vi "Program_EBN_Yann_Berton.vi"() -> ()   [LabVIEW 2020]
uses:
  Control Power/Commande.ctl
  <instrlib>/Keithley 27XX/Public/Configure/Measurement Specific/Configure Thermocouple.vi
  <instrlib>/Keithley 27XX/Public/Configure/Measurement Specific/Configure FRTD.vi
  <vilib>/Instr/_visa.llb/VISA Configure Serial Port (Instr).vi
  <instrlib>/Keithley 27XX/Keithley 27XX.lvlib
panel:
  in  "Number of samples allowed":dbl=15.0
  out "Close 50 mbar valve":bool
  out "T_ts_in_mid (wall)":dbl
  out "T_ts_in_top (wall)":dbl
  out "T_out_ts_mid (wall)":dbl
  out "T_out_ts_bot (wall)":dbl
  out "q_flux_TS (W/m²)":dbl
  out "Q_el TS (W)":dbl format="%_3g"
  out "Q_el PH (W)":dbl format="%_3g"
  in  "relative losses TS":dbl step=0.1
  in  "U Level TS":dbl step=0.1
  in  "STOP TS":bool
  out "Message 2":string
  out "Actual Voltage Level (V) TS":dbl format="%.3f"
  out "Actual Current Level (A) TS":dbl format="%.3f"
  out "status SGA":bool
  out "Power_Test section (W)":dbl format="%_3g"
  out "Warning_Temp_TS":bool
  in  "T limit_TS (C)":dbl=60.0 format="%#_13g"
  out "Temp max TS":dbl
  in  "U limit TS":dbl=8.0
  in  "I Limit TS":dbl=100.0
  out "error out 2":errorcluster caption="error out"
  in  "Power TS":bool
  out "Booléen 2":bool
  in  "relative losses PH":dbl step=0.1
  out "Counter":dbl
  out "T_PH_surf4":dbl
  out "T_PH_surf3":dbl
  out "TCHF_bot":dbl
  out "TCHF_top":dbl
  out "T3_bot":dbl
  out "T3_mid":dbl
  out "T3_top":dbl
  out "T2_top":dbl
  out "T2_mid":dbl
  out "T2_bot":dbl
  out "T1_top":dbl
  out "T1_mid":dbl
  out "T1_bot":dbl
  out "Pump cavitation":bool
  out "T_PH_surf2":dbl
  out "V_TS_corr (volts)":dbl
  out "V_PH_corr (volts)":dbl
  out "G (kg/m²s)":dbl
  out "x_out_TS":dbl
  out "x_in_TS":dbl
  out "i_in_ph":dbl
  out "i_v_TS_in":dbl
  out "i_l_TS_in":dbl
  out "T_sat(°C)":dbl
  in  "Fluid: 0 R1234ze; 1 R1233zd(E)":dbl
  out "Mass alert":bool
  in  "G minimum (kg/m²s)":dbl=20.0 format="%#_13g"
  out "Absolute pressure":dynamicdata(graph)
  out "Pressure drop":dynamicdata(graph)
  out "Temperatures":dynamicdata(graph)
  out "Temp max PH":dbl
  in  "T limit PH (C)":dbl=60.0 format="%#_13g"
  in  "STOP PH":bool
  out "Message":string
  out "Actual Voltage Level (V) PH":dbl format="%.3f"
  out "Actual Current Level (A) PH":dbl format="%.3f"
  out "Status DCS":bool
  out "Power_PRE HEATER (W)":dbl format="%_3g"
  in  "U limit PH":dbl=8.0
  in  "I Limit PH":dbl=100.0
  out "error out":errorcluster
  in  "U Level PH":dbl step=0.1
  in  "Power PH":bool
  out "Booléen":bool
  out "Warning_TEMP":bool
  in  "Porta RS232 Keithley 2701":refnum<visa-resource-name>="COM1"
  in  "Aquisition {Sample/s]":u32=1
  in  "stop":bool
  out "stop flag":bool
  out "V_TS_corr2":dbl
  out "P_reservoir (kPa)":dbl
  out "P_TS_in (kPa)":dbl
  out "P_pump_in (kPa)":dbl
  out "mass (kg/s)":dbl
  out "0-50 mbar (kPa)":dbl
  out "0-2 bar (kPa)":dbl
  out "T_ph_in (imm)":dbl
  out "T_amb":dbl
  out "T_reserv_bot":dbl
  out "T_reser_top":dbl
  out "T_TS_out_top (wall)":dbl
  out "T_TS_out (imm)":dbl
  out "T_PH_surf1":dbl
  out "T_PH_in (wall)":dbl
  out "T_TS_in (imm)":dbl
  out "T_TS_in_bot (wall)":dbl
  out "T_pump_in":dbl
  in  "File":path=path "C:/test.lvm" caption="Filename"
  in  "Save":bool caption="Enable"
  out "0-5 bar (kPa)":dbl
  out "Tcj ch201":dbl
  # "SAVING DATA"
  # "SGA Power supply: TEST SECTION POWER"
  # "DCS Power supply: PRE-HEATER POWER"
  # "Pre-heater temperatures"
  # "Test section temperatures"
  # "85 mm mm"
  # "40 mm"
  # "62.5 mm mm"
  # "665 mm"
  # "1347 mm mm"
  # "115 mm mm"
  # "809 mm"
  # "1585 mm mm"
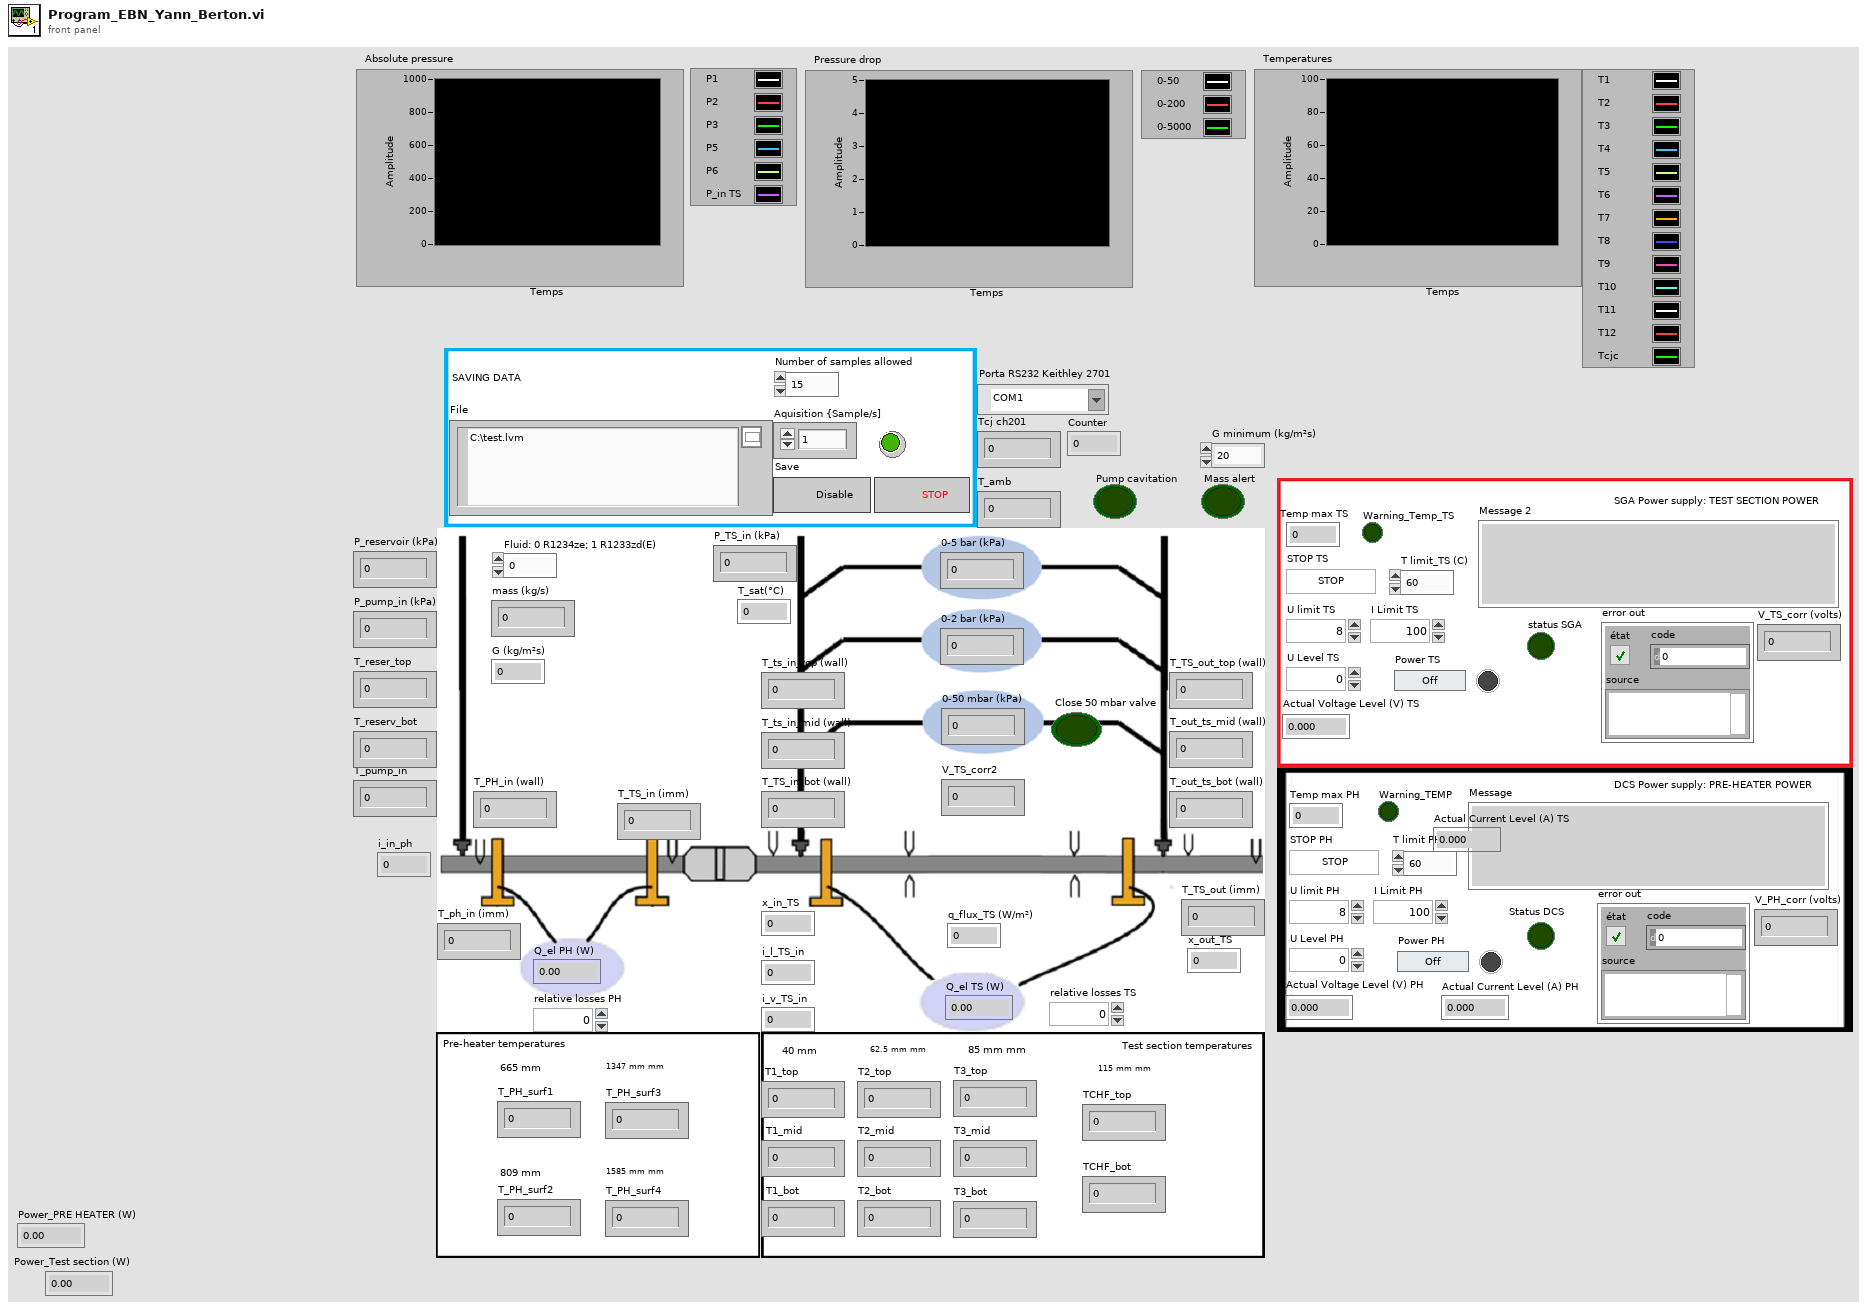
[diagram p1: front panel]
types:
  T1 = typedef "Commande.ctl" = enum16{"Power ON/OFF", "WaitForEvent", "Limit U&I", "Send ui", "Send U", "Meas", "Stop", "Init"}
  T2 = cluster{"Baud Rate (9600)":u32, "Flow Control (1: XON/XOFF)":u16, "Termination Char (0:CR)":u16}
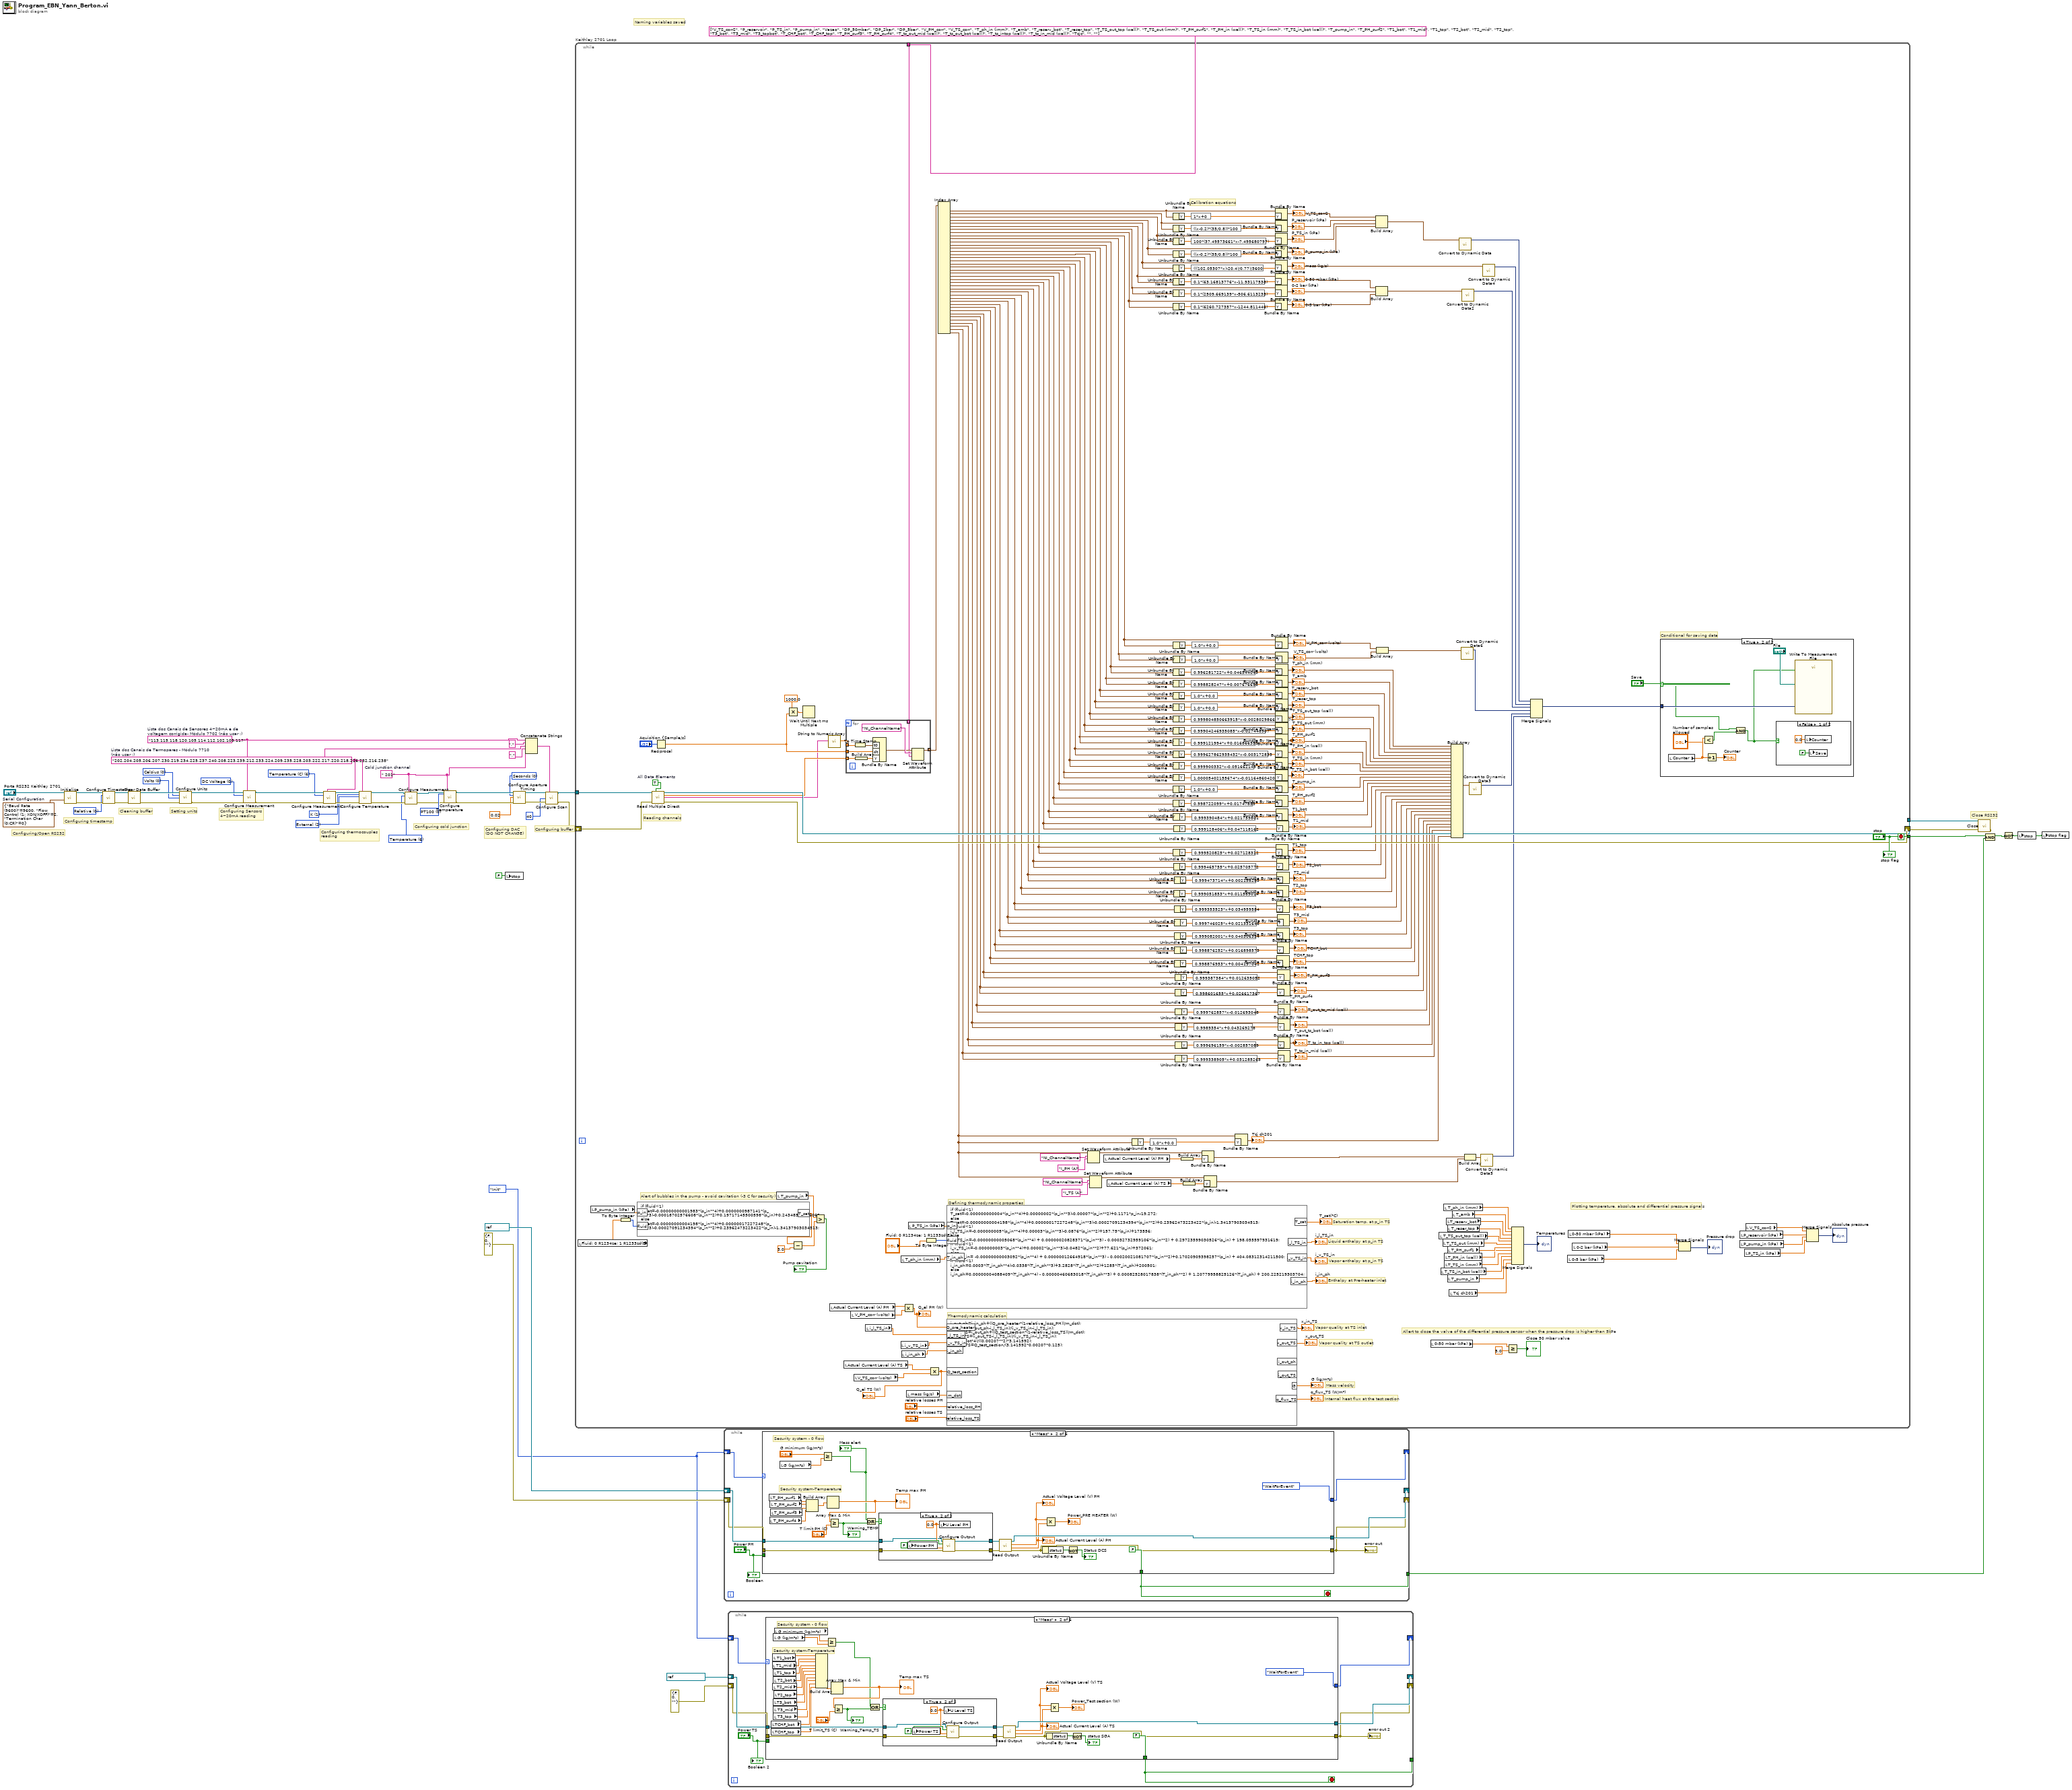
[diagram p0: block diagram]
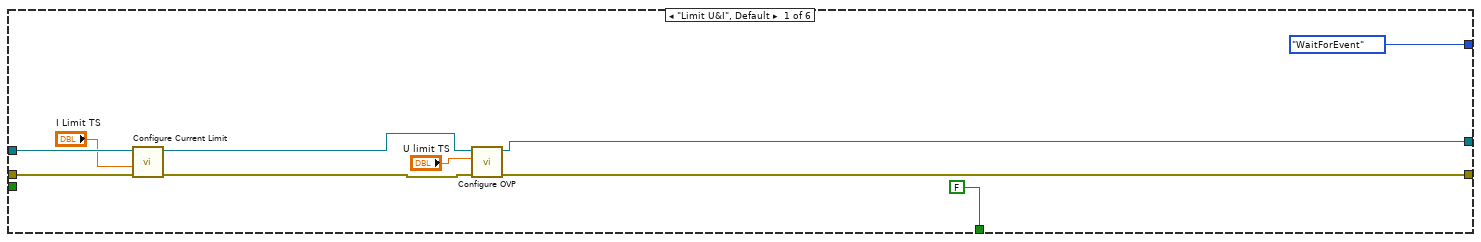
[diagram p2: hidden frame]
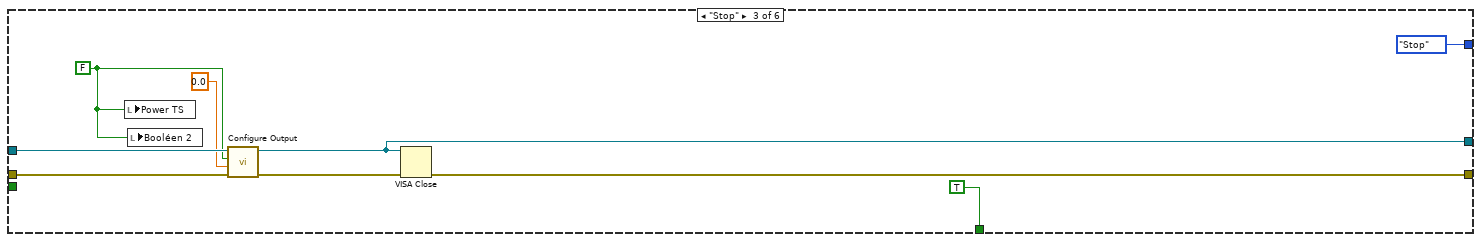
[diagram p4: hidden frame]
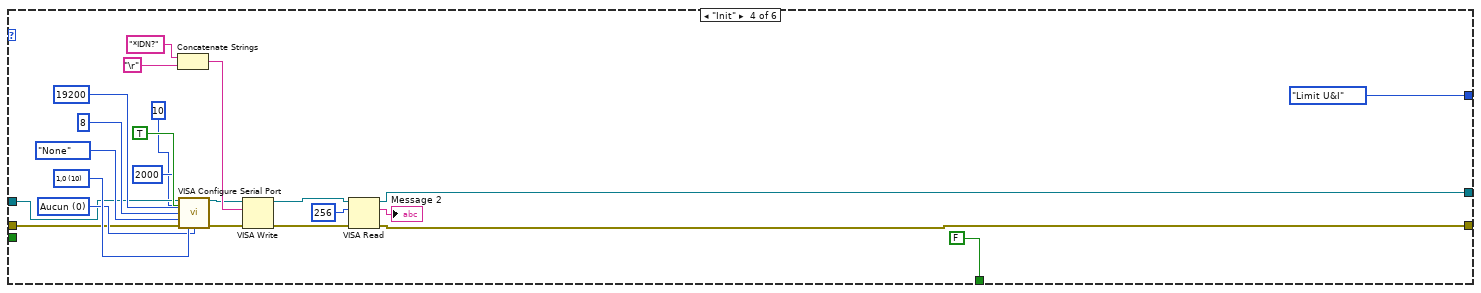
[diagram p5: hidden frame]
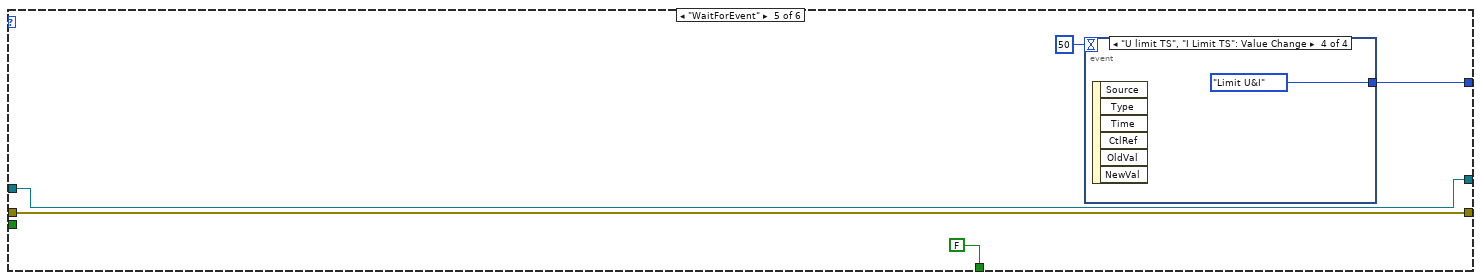
[diagram p6: hidden frame]
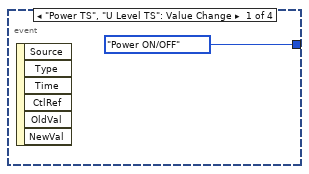
[diagram p7: hidden frame]
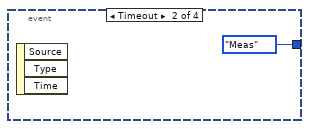
[diagram p8: hidden frame]
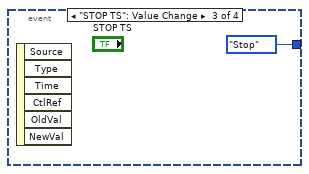
[diagram p9: hidden frame]
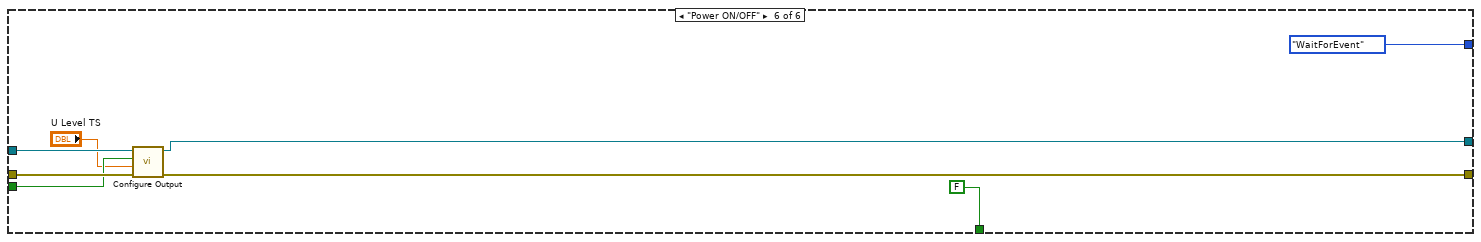
[diagram p10: hidden frame]
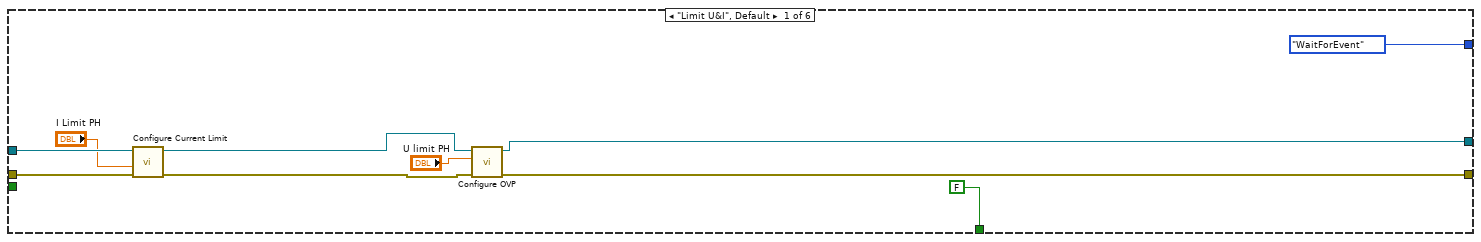
[diagram p11: hidden frame]
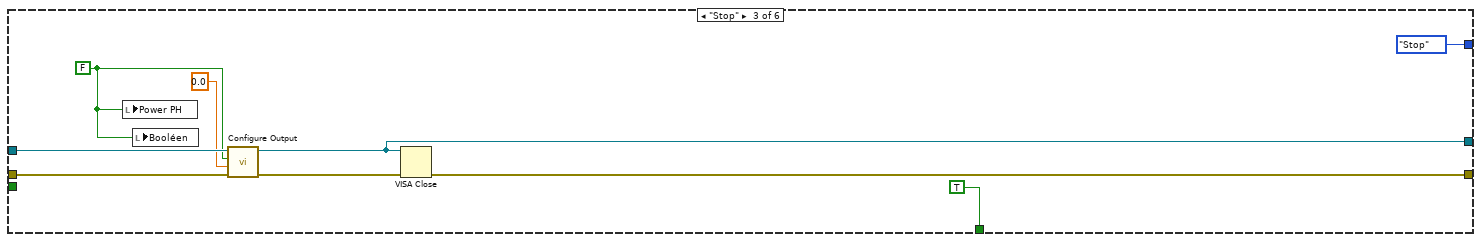
[diagram p13: hidden frame]
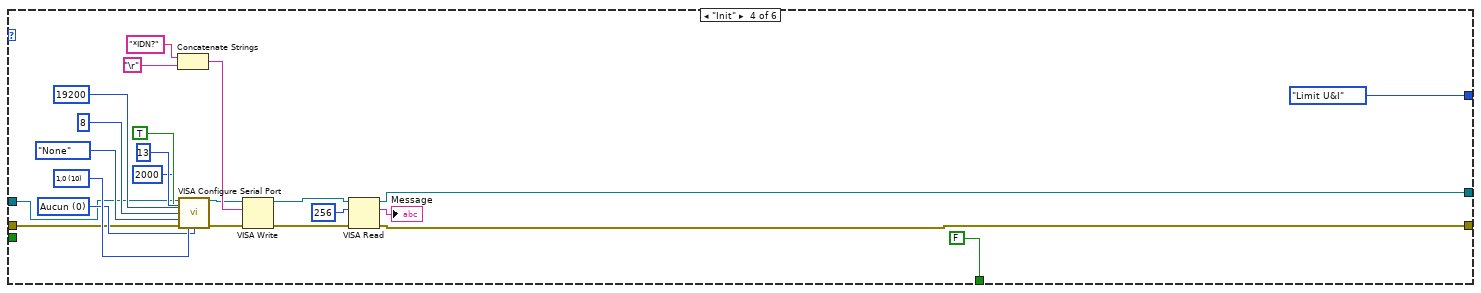
[diagram p14: hidden frame]
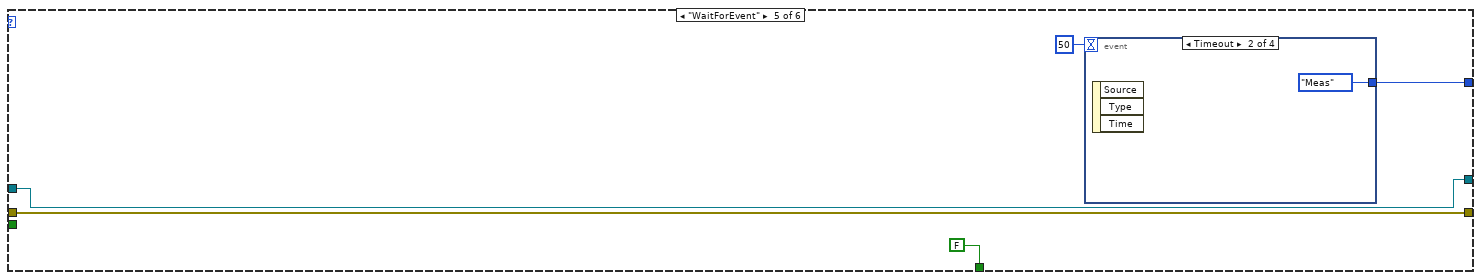
[diagram p15: hidden frame]
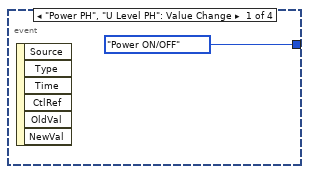
[diagram p16: hidden frame]
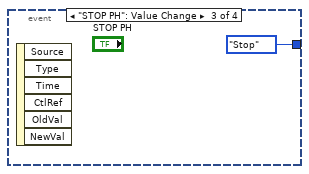
[diagram p17: hidden frame]
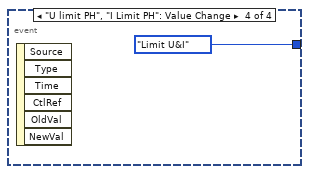
[diagram p18: hidden frame]
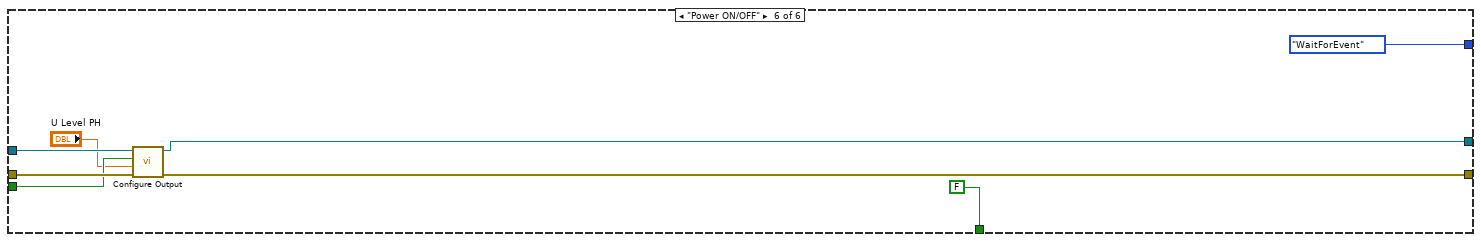
[diagram p19: hidden frame]
diagram:
  w3 = Commande."Init"
  w23 = u16 0 items=["PT100", "D100", "F100", "PT3916", "PT385", "USER"] ("FRTD Type (0: PT100)")
  w26 = u16 6 items=["DC Voltage", "AC Voltage", "DC Current", "AC Current", "Resistance", "Four-Wire Resistance", "Temperature", "Frequency", "Period", "Continuity"] ("Function (0: DC Voltage)")
  w24 = " 201"  # Cold junction channel
  w32 = "202,204,205,206,207,230,219,234,225,237,240,208,223,239,212,233,224,209,235,228,203,222,217,220,218,226,232,216,238"  # Lista dos Canais de Termopares - Módulo 7710 (não usar :)
  w40 = "113,115,118,120,105,114,112,102,109,117"  # Lista dos Canais de Sensores 4~20mA e de voltagem corrigida- Módulo 7702 (não usar :)
  w19 = u16 0 items=["Seconds", "Power Line Cycles"] ("Timing Units (0: Seconds)")
  w29 = u16 2 items=["Simulated", "Internal", "External"] ("Reference Junction Type (0: Simulated)")
  w30 = u16 1 items=["J", "K", "T", "E", "R", "S", "B", "N"] ("Thermocouple Type (1: K)")
  w41 = u16 0 items=["Volts", "dB"] ("DC Voltage (0: V)")
  w42 = u16 0 items=["Celsius", "Fahrenheit", "Kelvin"] ("Temperature (0: Celsius)")
  w34 = u16 6 items=["DC Voltage", "AC Voltage", "DC Current", "AC Current", "Resistance", "Four-Wire Resistance", "Temperature (C)", "Frequency", "Period", "Continuity"] ("Function (0: DC Voltage)")
  w37 = u16 0 items=["DC Voltage", "AC Voltage", "DC Current", "AC Current", "Resistance", "Four-Wire Resistance", "Temperature (C)", "Frequency", "Period", "Continuity"] ("Function (0: DC Voltage)")
  w50 = T2 {"Baud Rate (9600)"=9600, "Flow Control (1: XON/XOFF)"=2, "Termination Char (0:CR)"=0}  # Serial Configuration
  w47 = u16 0 items=["Relative", "Real Time Clock"] ("Timestamp Type (0: Relative)")
  # "Configuring cold junction"
  # "Naming variables saved"
  # "Close RS232"
  # "Configuring buffer"
  # "Configuring DAC \n(DO NOT CHANGE)"
  # "Configuring thermocouples\nreading"
  # "Configuring Sensors \n4~20mA reading"
  # "Setting units"
  # "Cleaning buffer"
  # "Configuring timestamp"
  # "Configuring/Open RS232"
  n1 = call <instrlib>:"Initialize.vi"("VISA resource name"="Porta RS232 Keithley 2701", "Serial Configuration"=w50) -> ("VISA resource name out"=w49:refnum<visa-resource-name>, "error out"=w48:errorcluster)  [unwired: 12 in]
  n2 = call <instrlib>:"Configure Timestamp.vi"("VISA resource name"=w49, "Timestamp Type (0: Relative)"=w47, "error in (no error)"=w48) -> ("VISA resource name out"=w46:refnum<visa-resource-name>, "error out"=w45:errorcluster)  [unwired: 11 in]
  n3 = call <instrlib>:"Clear Data Buffer.vi"("VISA resource name"=w46, "error in (no error)"=w45) -> ("VISA resource name out"=w44:refnum<visa-resource-name>, "error out"=w43:errorcluster)  [unwired: 12 in]
  n4 = call <instrlib>:"Configure Units.vi"("VISA resource name"=w44, "Temperature (0: Celsius)"=w42, "DC Voltage (0: V)"=w41, "error in (no error)"=w43) -> ("VISA resource name out"=w38:refnum<visa-resource-name>, "error out"=w39:errorcluster)  [unwired: 10 in]
  n5 = call <instrlib>:"Configure Measurement.vi"("VISA resource name"=w38, "Scan List (Empty)"=w40, "Function (0: DC Voltage)"=w37, "error in (no error)"=w39) -> ("VISA resource name out"=w36:refnum<visa-resource-name>, "error out"=w35:errorcluster)  [unwired: 10 in]
  n6 = call <instrlib>:"Configure Measurement.vi"("VISA resource name"=w36, "Scan List (Empty)"=w32, "Function (0: DC Voltage)"=w34, "error in (no error)"=w35) -> ("VISA resource name out"=w33:refnum<visa-resource-name>, "error out"=w31:errorcluster)  [unwired: 10 in]
  n7 = call-poly <instrlib>:"Configure Temperature.vi"("VISA resource name"=w33, "Thermocouple Type (1: K)"=w30, "Reference Junction Type (0: Simulated)"=w29, "error in (no error)"=w31, "Scan List (Empty)"=w32) -> ("VISA resource name out"=w28:refnum<visa-resource-name>, "error out"=w27:errorcluster)  [unwired: 13 in]
  n8 = call <instrlib>:"Configure Measurement.vi"("VISA resource name"=w28, "Scan List (Empty)"=w24, "Function (0: DC Voltage)"=w26, "error in (no error)"=w27) -> ("VISA resource name out"=w25:refnum<visa-resource-name>, "error out"=w22:errorcluster)  [unwired: 10 in]
  n9 = call-poly <instrlib>:"Configure Temperature.vi"("VISA resource name"=w25, "FRTD Type (0: PT100)"=w23, "error in (no error)"=w22, "Scan List (Empty)"=w24) -> ("VISA resource name out"=w21:refnum<visa-resource-name>, "error out"=w20:errorcluster)  [unwired: 14 in]
  n10 = local write "stop"(FALSE ("stop")) -> ()
  n11 = call <instrlib>:"Configure Aperture Timing.vi"("VISA resource name"=w21, "Timing Units (0: Seconds)"=w19, "Timing Value (0.020)"=0.02, "error in (no error)"=w20) -> ("VISA resource name out"=w16:refnum<visa-resource-name>, "error out"=w15:errorcluster)  [unwired: 10 in]
  n12 = Concatenate Strings(w40, "," ("string"), w32, "," ("string"), w24) -> (w17:string)
  n13 = call <instrlib>:"Configure Scan.vi"("VISA resource name"=w16, "Channel List (101:110)"=w17, "Sample Count (100)"=40 ("Sample Count (10)"), "error in (no error)"=w15) -> ("VISA resource name out"=w13:refnum<visa-resource-name>, "error out"=w14:errorcluster)  [unwired: 10 in]
  n14 = while "Keithley 2701 Loop" {
    tunnel: w13 -> [w257]
    tunnel: [w254] -> w11
    shift-right: [w255] -> w10
    shift-left: w14 -> [w256]
    tunnel: string[] ["V_TS_corr2", "P_reservoir", "P_TS_in", "P_pump_in", "Vazao", "DP_50mbar", "DP_2bar", "DP_5bar", "V_PH_corr", "V_TS_corr", "T_ph_in (imm)", "T_amb", "T_reserv_bot", "T_reser_top", "T_TS_out_top (wall)", "T_TS_out (imm)", "T_PH_surf1", "T_PH_in (wall)", "T_TS_in (imm)", "T_TS_in_bot (wall)", "T_pump_in", "T_PH_surf2", "T1_bot", "T1_mid", "T1_top", "T2_bot", "T2_mid", "T2_top", "T3_bot", "T3_mid", "T3_topbot", "T_CHF_bot", "T_CHF_top", "T_PH_surf3", "T_PH_surf4", "T_ts_out_mid (wall)", "T_ts_out_bot (wall)", "T_ts_intop (wall)", "T_ts_in_mid (wall)", "Tcjc", "", ""] -> [w308]
    tunnel: ["stop"] -> w7
    stop <- "stop" stop-if-true
    w250 = TRUE  # All Data Elements
    # "Allert to close the valve of the differential pressure sensor when the pressure drop is higher than 5kPa"
    # "Internal heat flux at the test section"
    # "Alert of bubbles in the pump - avoid cavitation (-3 C for security)"
    # "Mass velocity"
    # "Vapor quality at TS outlet"
    # "Vapor quality at TS inlet"
    # "Thermodynamic calculation"
    # "Enthalpy at Pre-heater inlet"
    # "Vapor enthalpy at p_in TS"
    # "Liquid enthalpy at p_in TS"
    # "Saturation temp. at p_in TS"
    # "Defining thermodynamic properties"
    # "Plotting temperature, absolute and differential pressure signals"
    # "Conditional for saving data"
    # "Calibration equations"
    # "Reading channels"
    n15 = local read "Fluid: 0 R1234ze; 1 R1233zd(E)"() -> (w166:dbl)
    n16 = local read "P_pump_in (kPa)"() -> (w172:dbl)
    n17 = To Byte Integer(number=w166) -> (8bit integer=w165:i8)
    n18 = formula code="if (fluid<1)\nT_sat=-0.00000000001983*(p_in**4)+0.0000000987141*(p_in**3)-0.00018702576608*(p_in**2)+0.19717145500598*(p_in)+0.24348535016065;\nelse\nT_sat=-0.00000000004198*(p_in**4)+0.00000017227248*(p_in**3)-0.00027091234394*(p_in**2)+0.23962473223422*(p_in)-1.34137903034513;"("p_in"=w172, "fluid"=w165) -> ("T_sat"=w168:dbl)
    n19 = call <instrlib>:"Read Multiple Direct.vi"("VISA resource name"=w257, "All Data Elements (False)"=w250, "error in (no error)"=w256) -> ("VISA resource name out"=w254:refnum<visa-resource-name>, "Measurement Data"=w253:dbl[], "Time Stamp"=w252:string[], "error out"=w255:errorcluster)  [unwired: 7 in, 2 out]
    n20 = Reciprocal(x="Aquisition {Sample/s]") -> (1/x=w309:dbl)
    n21 = local read "T_pump_in"() -> (w171:dbl)
    n22 = Multiply(x=1000.0 ("y"), y=w309) -> (x*y=w310:dbl)
    n23 = Subtract(x=w168, y=3.0) -> (x-y=w167:dbl)
    n24 = Wait Until Next ms Multiple(millisecond multiple=w310) -> ()  [unwired: 1 out]
    n25 = Greater?(x=w171, y=w167) -> (0:→"Pump cavitation":bool)
    n26 = call <instrlib>:"String to Numeric Array.vi"("String Array"=w252) -> ("Numeric Array"=w251:dbl[])  [unwired: 10 in]
    n27 = local read "Actual Current Level (A) PH"() -> (w89:dbl)
    n28 = local read "Actual Current Level (A) TS"() -> (w85:dbl)
    n29 = for {
      tunnel: w251 -> [w331] mode=indexing
      tunnel: w253 -> [w329] mode=indexing
      tunnel: w309 -> [w327]
      tunnel: w308 -> [w324] mode=indexing
      tunnel: [w323] -> w307 mode=indexing
      n30 = To Time Stamp(1:w331) -> (0:w330:timestamp)
      n31 = Build Array(w329) -> (w328:dbl[])
      n32 = Bundle By Name("t0"=w330, "dt"=w327, "Y"=w328) -> (w325:waveform(dbl))  [unwired: 1 in]
      n33 = Set Waveform Attribute(5:w324, 6:"NI_ChannelName" ("name"), 7:w325) -> (3:w323:waveform(dbl))  [unwired: 1 in, 2 out]
    }
    n34 = local read "V_PH_corr (volts)"() -> (w88:dbl)
    n35 = local read "V_TS_corr (volts)"() -> (w86:dbl)
    n36 = local read "i_l_TS_in"() -> (w58:dbl)
    n37 = local read "i_v_TS_in"() -> (w57:dbl)
    n38 = local read "T_ph_in (imm)"() -> (w212:dbl)
    n39 = local read "i_in_ph"() -> (w56:dbl)
    n40 = Multiply(x=w89, y=w88) -> (x*y=w87:dbl)
    "Q_el PH (W)" <- w87
    n41 = local read "mass (kg/s)"() -> (w164:dbl)
    n42 = local read "P_TS_in (kPa)"() -> (w214:dbl)
    n43 = To Byte Integer(number="Fluid: 0 R1234ze; 1 R1233zd(E)") -> (8bit integer=w205:i8)
    n44 = Multiply(x=w85, y=w86) -> (x*y=w83:dbl)
    "Q_el TS (W)" <- w83
    n45 = Index Array(array=w307) -> (element #1=w200:waveform(dbl), element #2=w199:waveform(dbl), element #3=w198:waveform(dbl), element #4=w197:waveform(dbl), element #5=w196:waveform(dbl), element #6=w195:waveform(dbl), element #7=w61:waveform(dbl), element #8=w194:waveform(dbl), element #9=w186:waveform(dbl), element #10=w183:waveform(dbl), element #11=w262:waveform(dbl), element #12=w263:waveform(dbl), element #13=w264:waveform(dbl), element #14=w265:waveform(dbl), element #15=w266:waveform(dbl), element #16=w267:waveform(dbl), element #17=w268:waveform(dbl), element #18=w269:waveform(dbl), element #19=w270:waveform(dbl), element #20=w271:waveform(dbl), element #21=w272:waveform(dbl), element #22=w173:waveform(dbl), element #23=w161:waveform(dbl), element #24=w156:waveform(dbl), element #25=w155:waveform(dbl), element #26=w148:waveform(dbl), element #27=w147:waveform(dbl), element #28=w146:waveform(dbl), element #29=w139:waveform(dbl), element #30=w138:waveform(dbl), element #31=w137:waveform(dbl), element #32=w132:waveform(dbl), element #33=w131:waveform(dbl), element #34=w94:waveform(dbl), element #35=w93:waveform(dbl), element #36=w77:waveform(dbl), element #37=w76:waveform(dbl), element #38=w71:waveform(dbl), element #39=w67:waveform(dbl), element #40=w59:waveform(dbl))  [unwired: 40 in]
    n46 = formula code="if (fluid<1)\nT_sat=-0.000000000004*(p_in**4)+0.00000002*(p_in**3)-0.00007*(p_in**2)+0.1171*p_in-19.272;\nelse\nT_sat=-0.00000000004198*(p_in**4)+0.00000017227248*(p_in**3)-0.00027091234394*(p_in**2)+0.23962473223422*(p_in)-1.34137903034513;\nif (fluid<1)\ni_l_TS_in=-0.000000005*(p_in**4)+0.00003*(p_in**3)-0.0876*(p_in**2)+157.75*(p_in)+173556;\nelse\ni_l_TS_in=-0.00000000005068*(p_in**4) + 0.00000020828371*(p_in**3) - 0.00032732959106*(p_in**2) + 0.29723599030526*(p_in) + 198.055597931619;\nif (fluid<1)\ni_v_TS_in=-0.000000003*(p_in**4)+0.00002*(p_in**3)-0.0482*(p_in**2)+77.621*(p_in)+372061;\nelse \ni_v_TS_in= -0.00000000003092*(p_in**4) + 0.00000012664918*(p_in**3) - 0.00020021081707*(p_in**2)+0.17020909398257*(p_in) + 404.08312314211500;\nif (fluid<1)\ni_in_ph=0.0003*(T_in_ph**4)-0.0338*(T_in_ph**3)+3.2828*(T_in_ph**2)+1285*(T_in_ph)+200501;\nelse\ni_in_ph=0.00000004088409*(T_in_ph**4) - 0.00000460683018*(T_in_ph**3) + 0.00082528017838*(T_in_ph**2) + 1.20779958825126*(T_in_ph) + 200.225219303704;"("p_in"=w214, "fluid"=w205, "T_in_ph"=w212) -> ("T_sat"=→"T_sat(°C)":dbl, "i_l_TS_in"=→"i_l_TS_in":dbl, "i_v_TS_in"=→"i_v_TS_in":dbl, "i_in_ph"=→"i_in_ph":dbl)
    n47 = formula code="i_out_ph=i_in_ph+((Q_pre_heater*(1-relative_loss_PH))/m_dot);\nx_in_TS=(i_out_ph-i_l_TS_in)/(i_v_TS_in-i_l_TS_in);\ni_out_TS=i_out_ph+((Q_test_section*(1-relative_loss_TS))/m_dot);\nx_out_TS=(i_out_TS-i_l_TS_in)/(i_v_TS_in-i_l_TS_in);\nG=(m_dot*4)/((0.00207**2)*3.141592);\nq_flux_TS=Q_test_section/(3.141592*0.00207*0.125);"("i_l_TS_in"=w58, "i_v_TS_in"=w57, "i_in_ph"=w56, "Q_pre_heater"=w87, "Q_test_section"=w83, "m_dot"=w164, "relative_loss_PH"="relative losses PH", "relative_loss_TS"="relative losses TS") -> ("x_in_TS"=→"x_in_TS":dbl, "x_out_TS"=→"x_out_TS":dbl, "G"=→"G (kg/m²s)":dbl, "q_flux_TS"=→"q_flux_TS (W/m²)":dbl)  [unwired: 2 out]
    n48 = Set Waveform Attribute(5:"I_PH (A)" ("name"), 6:"NI_ChannelName" ("name"), 7:w59) -> (3:w247:waveform(dbl))  [unwired: 1 in, 2 out]
    n49 = Set Waveform Attribute(5:"I_TS (A)" ("name"), 6:"NI_ChannelName" ("name"), 7:w59) -> (3:w102:waveform(dbl))  [unwired: 1 in, 2 out]
    n50 = local read "Actual Current Level (A) PH"() -> (w177:dbl)
    n51 = local read "Actual Current Level (A) TS"() -> (w104:dbl)
    n52 = Unbundle By Name(w59) -> ("Y"=w261:dbl[])
    n53 = expression code="1.0*x+0.0"(w261) -> (w232:dbl[])
    n54 = Unbundle By Name(w200) -> ("Y"=w305:dbl[])
    n55 = Unbundle By Name(w199) -> ("Y"=w302:dbl[])
    n56 = Unbundle By Name(w198) -> ("Y"=w304:dbl[])
    n57 = Unbundle By Name(w197) -> ("Y"=w297:dbl[])
    n58 = Unbundle By Name(w196) -> ("Y"=w301:dbl[])
    n59 = Unbundle By Name(w195) -> ("Y"=w298:dbl[])
    n60 = Unbundle By Name(w61) -> ("Y"=w295:dbl[])
    n61 = Unbundle By Name(w194) -> ("Y"=w274:dbl[])
    n62 = Unbundle By Name(w262) -> ("Y"=w293:dbl[])
    n63 = Unbundle By Name(w263) -> ("Y"=w291:dbl[])
    n64 = Unbundle By Name(w264) -> ("Y"=w292:dbl[])
    n65 = Unbundle By Name(w265) -> ("Y"=w287:dbl[])
    n66 = Unbundle By Name(w266) -> ("Y"=w288:dbl[])
    n67 = Unbundle By Name(w267) -> ("Y"=w290:dbl[])
    n68 = Unbundle By Name(w268) -> ("Y"=w289:dbl[])
    n69 = Unbundle By Name(w269) -> ("Y"=w283:dbl[])
    n70 = Unbundle By Name(w270) -> ("Y"=w286:dbl[])
    n71 = Unbundle By Name(w271) -> ("Y"=w285:dbl[])
    n72 = Unbundle By Name(w272) -> ("Y"=w284:dbl[])
    n73 = Unbundle By Name(w173) -> ("Y"=w175:dbl[])
    n74 = Unbundle By Name(w186) -> ("Y"=w188:dbl[])
    n75 = Unbundle By Name(w183) -> ("Y"=w184:dbl[])
    n76 = Unbundle By Name(w161) -> ("Y"=w162:dbl[])
    n77 = Unbundle By Name(w155) -> ("Y"=w157:dbl[])
    n78 = Unbundle By Name(w156) -> ("Y"=w160:dbl[])
    n79 = Unbundle By Name(w148) -> ("Y"=w154:dbl[])
    n80 = Unbundle By Name(w146) -> ("Y"=w150:dbl[])
    n81 = Unbundle By Name(w147) -> ("Y"=w152:dbl[])
    n82 = Unbundle By Name(w139) -> ("Y"=w140:dbl[])
    n83 = Unbundle By Name(w137) -> ("Y"=w144:dbl[])
    n84 = Unbundle By Name(w131) -> ("Y"=w134:dbl[])
    n85 = Unbundle By Name(w138) -> ("Y"=w142:dbl[])
    n86 = Unbundle By Name(w132) -> ("Y"=w136:dbl[])
    n87 = Unbundle By Name(w94) -> ("Y"=w98:dbl[])
    n88 = Unbundle By Name(w93) -> ("Y"=w96:dbl[])
    n89 = Unbundle By Name(w77) -> ("Y"=w78:dbl[])
    n90 = Unbundle By Name(w76) -> ("Y"=w80:dbl[])
    n91 = Unbundle By Name(w71) -> ("Y"=w73:dbl[])
    n92 = Unbundle By Name(w67) -> ("Y"=w68:dbl[])
    n93 = Build Array(w177) -> (w246:dbl[])
    n94 = Build Array(w104) -> (w103:dbl[])
    n95 = expression code="1*x+0"(w305) -> (w306:dbl[])
    n96 = expression code="((x-0.2)*(35/0.8))*100"(w302) -> (w303:dbl[])
    n97 = expression code="100*(37.49573661*x-7.495680797)"(w304) -> (w260:dbl[])
    n98 = expression code="((x-0.2)*(35/0.8))*100"(w297) -> (w296:dbl[])
    n99 = expression code="(((102.05307*x)-20.4)/0.77)/3600"(w301) -> (w300:dbl[])
    n100 = expression code="0.1*(63.16813776*x-11.93117538)"(w298) -> (w299:dbl[])
    n101 = expression code="0.1*(2509.669139*x-506.6113235)"(w295) -> (w294:dbl[])
    n102 = expression code="0.1*(6260.727357*x-1244.811446)"(w274) -> (w275:dbl[])
    n103 = expression code="0.996281722*x+0.046544049"(w293) -> (w233:dbl[])
    n104 = expression code="0.998828247*x+0.007676698"(w291) -> (w234:dbl[])
    n105 = expression code="1.0*x+0.0"(w292) -> (w244:dbl[])
    n106 = expression code="1.0*x+0.0"(w287) -> (w243:dbl[])
    n107 = expression code="0.999804850663915*x-0.00280298667172474"(w288) -> (w242:dbl[])
    n108 = expression code="0.99904246935085*x-0.027448907"(w290) -> (w241:dbl[])
    n109 = expression code="0.999121994*x+0.016866359"(w289) -> (w240:dbl[])
    n110 = expression code="0.999627862935432*x-0.003172835"(w283) -> (w239:dbl[])
    n111 = expression code="0.999900332*x-0.051662145"(w286) -> (w238:dbl[])
    n112 = expression code="1.00005402155674*x-0.0116486042091708"(w285) -> (w237:dbl[])
    n113 = expression code="1.0*x+0.0"(w284) -> (w236:dbl[])
    n114 = expression code="0.998722099*x+0.01747855"(w175) -> (w174:dbl[])
    n115 = expression code="1.0*x+0.0"(w188) -> (w187:dbl[])
    n116 = expression code="1.0*x+0.0"(w184) -> (w185:dbl[])
    n117 = expression code="0.999390484*x+0.021759801"(w162) -> (w163:dbl[])
    n118 = expression code="0.999520825*x+0.027128312"(w157) -> (w158:dbl[])
    n119 = expression code="0.999128406*x+0.047118162"(w160) -> (w159:dbl[])
    n120 = expression code="0.999465755*x+0.025705772"(w154) -> (w153:dbl[])
    n121 = expression code="0.999051853*x+0.011589014"(w150) -> (w149:dbl[])
    n122 = expression code="0.999473714*x+0.002158285"(w152) -> (w151:dbl[])
    n123 = expression code="0.999353523*x+0.034959584"(w140) -> (w141:dbl[])
    n124 = expression code="0.999082001*x+0.040306354"(w144) -> (w145:dbl[])
    n125 = expression code="0.998876953*x+0.004197041"(w134) -> (w133:dbl[])
    n126 = expression code="0.999746025*x+0.021331648"(w142) -> (w143:dbl[])
    n127 = expression code="0.998876252*x+0.016898573"(w136) -> (w135:dbl[])
    n128 = expression code="0.999387384*x+0.012635052"(w98) -> (w97:dbl[])
    n129 = expression code="0.998601655*x+0.026617367"(w96) -> (w95:dbl[])
    n130 = expression code="0.999762857*x-0.012693048"(w78) -> (w79:dbl[])
    n131 = expression code="0.9989354*x+0.043269278"(w80) -> (w81:dbl[])
    n132 = expression code="0.999696159*x-0.002857089"(w73) -> (w72:dbl[])
    n133 = expression code="0.999338905*x+0.031285265"(w68) -> (w69:dbl[])
    n134 = Bundle By Name(cluster=w247, "Y"=w246) -> (w105:waveform(dbl))
    n135 = Bundle By Name(cluster=w102, "Y"=w103) -> (w99:waveform(dbl))
    n136 = Bundle By Name(cluster=w59, "Y"=w232) -> (w60:waveform(dbl))
    "Tcj ch201" <- w60
    n137 = Bundle By Name(cluster=w200, "Y"=w306) -> (w204:waveform(dbl))
    "V_TS_corr2" <- w204
    n138 = Bundle By Name(cluster=w199, "Y"=w303) -> (w203:waveform(dbl))
    "P_reservoir (kPa)" <- w203
    n139 = Bundle By Name(cluster=w198, "Y"=w260) -> (w202:waveform(dbl))
    "P_TS_in (kPa)" <- w202
    n140 = Bundle By Name(cluster=w197, "Y"=w296) -> (w201:waveform(dbl))
    "P_pump_in (kPa)" <- w201
    n141 = Bundle By Name(cluster=w196, "Y"=w300) -> (w259:waveform(dbl))
    "mass (kg/s)" <- w259
    n142 = Bundle By Name(cluster=w195, "Y"=w299) -> (w63:waveform(dbl))
    "0-50 mbar (kPa)" <- w63
    n143 = Bundle By Name(cluster=w61, "Y"=w294) -> (w278:waveform(dbl))
    "0-2 bar (kPa)" <- w278
    n144 = Bundle By Name(cluster=w194, "Y"=w275) -> (w273:waveform(dbl))
    "0-5 bar (kPa)" <- w273
    n145 = Bundle By Name(cluster=w186, "Y"=w187) -> (w180:waveform(dbl))
    "V_PH_corr (volts)" <- w180
    n146 = Bundle By Name(cluster=w183, "Y"=w185) -> (w179:waveform(dbl))
    "V_TS_corr (volts)" <- w179
    n147 = Bundle By Name(cluster=w262, "Y"=w233) -> (w130:waveform(dbl))
    "T_ph_in (imm)" <- w130
    n148 = Bundle By Name(cluster=w263, "Y"=w234) -> (w129:waveform(dbl))
    "T_amb" <- w129
    n149 = Bundle By Name(cluster=w264, "Y"=w244) -> (w128:waveform(dbl))
    "T_reserv_bot" <- w128
    n150 = Bundle By Name(cluster=w265, "Y"=w243) -> (w127:waveform(dbl))
    "T_reser_top" <- w127
    n151 = Bundle By Name(cluster=w266, "Y"=w242) -> (w126:waveform(dbl))
    "T_TS_out_top (wall)" <- w126
    n152 = Bundle By Name(cluster=w267, "Y"=w241) -> (w125:waveform(dbl))
    "T_TS_out (imm)" <- w125
    n153 = Bundle By Name(cluster=w268, "Y"=w240) -> (w124:waveform(dbl))
    "T_PH_surf1" <- w124
    n154 = Bundle By Name(cluster=w269, "Y"=w239) -> (w123:waveform(dbl))
    "T_PH_in (wall)" <- w123
    n155 = Bundle By Name(cluster=w270, "Y"=w238) -> (w122:waveform(dbl))
    "T_TS_in (imm)" <- w122
    n156 = Bundle By Name(cluster=w271, "Y"=w237) -> (w121:waveform(dbl))
    "T_TS_in_bot (wall)" <- w121
    n157 = Bundle By Name(cluster=w272, "Y"=w236) -> (w120:waveform(dbl))
    "T_pump_in" <- w120
    n158 = Bundle By Name(cluster=w173, "Y"=w174) -> (w119:waveform(dbl))
    "T_PH_surf2" <- w119
    n159 = Bundle By Name(cluster=w161, "Y"=w163) -> (w118:waveform(dbl))
    "T1_bot" <- w118
    n160 = Bundle By Name(cluster=w155, "Y"=w158) -> (w116:waveform(dbl))
    "T1_top" <- w116
    n161 = Bundle By Name(cluster=w156, "Y"=w159) -> (w117:waveform(dbl))
    "T1_mid" <- w117
    n162 = Bundle By Name(cluster=w148, "Y"=w153) -> (w115:waveform(dbl))
    "T2_bot" <- w115
    n163 = Bundle By Name(cluster=w146, "Y"=w149) -> (w113:waveform(dbl))
    "T2_top" <- w113
    n164 = Bundle By Name(cluster=w147, "Y"=w151) -> (w114:waveform(dbl))
    "T2_mid" <- w114
    n165 = Bundle By Name(cluster=w139, "Y"=w141) -> (w112:waveform(dbl))
    "T3_bot" <- w112
    n166 = Bundle By Name(cluster=w137, "Y"=w145) -> (w110:waveform(dbl))
    "T3_top" <- w110
    n167 = Bundle By Name(cluster=w131, "Y"=w133) -> (w108:waveform(dbl))
    "TCHF_top" <- w108
    n168 = Bundle By Name(cluster=w138, "Y"=w143) -> (w111:waveform(dbl))
    "T3_mid" <- w111
    n169 = Bundle By Name(cluster=w132, "Y"=w135) -> (w109:waveform(dbl))
    "TCHF_bot" <- w109
    n170 = Bundle By Name(cluster=w94, "Y"=w97) -> (w92:waveform(dbl))
    "T_PH_surf3" <- w92
    n171 = Bundle By Name(cluster=w93, "Y"=w95) -> (w91:waveform(dbl))
    "T_PH_surf4" <- w91
    n172 = Bundle By Name(cluster=w77, "Y"=w79) -> (w75:waveform(dbl))
    "T_out_ts_mid (wall)" <- w75
    n173 = Bundle By Name(cluster=w76, "Y"=w81) -> (w74:waveform(dbl))
    "T_out_ts_bot (wall)" <- w74
    n174 = Bundle By Name(cluster=w71, "Y"=w72) -> (w70:waveform(dbl))
    "T_ts_in_top (wall)" <- w70
    n175 = Bundle By Name(cluster=w67, "Y"=w69) -> (w66:waveform(dbl))
    "T_ts_in_mid (wall)" <- w66
    n176 = Build Array(w204, w203, w202, w201) -> (w245:waveform(dbl)[])
    n177 = Build Array(w63, w278, w273) -> (w282:waveform(dbl)[])
    n178 = Build Array(w180, w179) -> (w181:waveform(dbl)[])
    n179 = local read "0-50 mbar (kPa)"() -> (w62:dbl)
    n180 = local read "T_TS_out_top (wall)"() -> (w226:dbl)
    n181 = local read "T_TS_in_bot (wall)"() -> (w222:dbl)
    n182 = local read "T_TS_out (imm)"() -> (w225:dbl)
    n183 = local read "T_ph_in (imm)"() -> (w230:dbl)
    n184 = local read "T_PH_in (wall)"() -> (w220:dbl)
    n185 = local read "T_TS_in (imm)"() -> (w221:dbl)
    n186 = local read "T_reserv_bot"() -> (w228:dbl)
    n187 = local read "T_reser_top"() -> (w227:dbl)
    n188 = local read "T_PH_surf1"() -> (w224:dbl)
    n189 = local read "T_pump_in"() -> (w223:dbl)
    n190 = local read "Tcj ch201"() -> (w176:dbl)
    n191 = Build Array(w130, w129, w128, w127, w126, w125, w124, w123, w122, w121, w120, w119, w118, w117, w116, w115, w114, w113, w112, w111, w110, w109, w108, w92, w91, w75, w74, w70, w66, w60) -> (w235:waveform(dbl)[])
    n192 = local read "T_amb"() -> (w229:dbl)
    n193 = call "Convert to Dynamic Data"("Array of Waveforms"=w245) -> ("Dynamic Data Type"=w279:dynamicdata)  [unwired: 3 in]
    n194 = call "Convert to Dynamic Data6"("Array of Waveforms"=w181) -> ("Dynamic Data Type"=w178:dynamicdata)  [unwired: 3 in]
    n195 = call "Convert to Dynamic Data2"("Array of Waveforms"=w282) -> ("Dynamic Data Type"=w280:dynamicdata)  [unwired: 3 in]
    n196 = Build Array(w105, w99) -> (w107:waveform(dbl)[])
    n197 = call "Convert to Dynamic Data3"("Array of Waveforms"=w235) -> ("Dynamic Data Type"=w182:dynamicdata)  [unwired: 3 in]
    n198 = call "Convert to Dynamic Data5"("Array of Waveforms"=w107) -> ("Dynamic Data Type"=w106:dynamicdata)  [unwired: 3 in]
    n199 = call "Convert to Dynamic Data4"("Waveform"=w259) -> ("Dynamic Data Type"=w258:dynamicdata)  [unwired: 3 in]
    n200 = Greater Or Equal?(x=w62, y=5.0) -> (x >= y?=→"Close 50 mbar valve":bool)
    n201 = Merge Signals(w230, w229, w228, w227, w226, w225, w224, w220, w221, w222, w223, w176) -> (→"Temperatures":dynamicdata)
    n202 = Merge Signals(w279, w258, w280, w178, w182, w106) -> (w281:dynamicdata)
    n203 = local read "0-5 bar (kPa)"() -> (w215:dbl)
    n204 = local read "0-50 mbar (kPa)"() -> (w217:dbl)
    n205 = local read "0-2 bar (kPa)"() -> (w216:dbl)
    n206 = case shown="True" "Save" {
      selector: "Save" -> [_ w316]
      tunnel: w281 -> [_ w320]
      frame False {
      }
      frame True {
        n207 = local read "Counter"() -> (w317:dbl)
        n208 = Less?(x=w317, y="Number of samples allowed") -> (x < y?=w315:bool)
        n209 = Increment(x=w317) -> (x+1=→"Counter":dbl)
        n210 = And(x=w316, y=w315) -> (x .and. y?=w314:bool)
        n211 = case shown="False" w314 {
          frame False {
            n212 = local write "Counter"(0.0 ("Counter")) -> ()
            n213 = local write "Save"(FALSE ("Save")) -> ()
          }
          frame True {
          }
        }
        n214 = call "Write To Measurement File"("Signals"=w320, "Enable"=w314, "Filename"="File") -> ()  [unwired: 14 in, 3 out]
      }
    }
    n215 = Merge Signals(w217, w216, w215) -> (→"Pressure drop":dynamicdata)
    n216 = local read "P_reservoir (kPa)"() -> (w192:dbl)
    n217 = local read "P_pump_in (kPa)"() -> (w191:dbl)
    n218 = local read "P_TS_in (kPa)"() -> (w190:dbl)
    n219 = local read "V_TS_corr2"() -> (w193:dbl)
    n220 = Merge Signals(w193, w192, w191, w190) -> (→"Absolute pressure":dynamicdata)
    "stop flag" <- "stop"
  }
  n221 = while {
    shift-right: [w338] -> _
    shift-left: w3 -> [w339]
    shift-right: [w337] -> _
    shift-left: refnum<visa-resource-name> "COM4" ("VISA resource name") -> [w335]
    shift-right: [w336] -> _
    shift-left: errorcluster {"status"=FALSE, "code"=0, "source"=""} ("error in (no error)") -> [w334]
    tunnel: [w333] -> w6
    stop <- w333 stop-if-true
    n222 = case shown="\"Meas\"" w339 {
      tunnel: [FALSE FALSE TRUE FALSE FALSE FALSE] -> w333
      tunnel: [Commande."WaitForEvent" Commande."WaitForEvent" Commande."Stop" Commande."Limit U&I" w419 Commande."WaitForEvent"] -> w338
      tunnel: [w342 w374 w385 w399 w416 w429] -> w337
      tunnel: [w341 w371 w389 w398 w417 w428] -> w336
      tunnel: w335 -> [w349 w364 w388 w397 w416 w431]
      tunnel: w334 -> [w348 w363 w387 w396 w417 w430]
      tunnel: "Power PH" -> [_ _ _ _ _ w425]
      frame "Limit U&I", Default {
        n223 = call "Configure Current Limit.vi"("error in (no error)"=w348, "Current Limit (0.00 A)"="I Limit PH", "VISA resource name"=w349) -> ("error out"=w343:errorcluster, "VISA resource name out"=w344:refnum<visa-resource-name>)  [unwired: 6 in, 1 out]
        n224 = call "Configure OVP.vi"("error in (no error)"=w343, "Overvoltage Protection Value (110.0 V)"="U limit PH", "VISA resource name"=w344) -> ("error out"=w341:errorcluster, "VISA resource name out"=w342:refnum<visa-resource-name>)  [unwired: 7 in]
      }
      frame "Meas" {
        # "Security system - 0 flow"
        # "Security system-Temperature"
        n225 = local read "T_PH_surf1"() -> (w357:dbl)
        n226 = local read "T_PH_surf4"() -> (w352:dbl)
        n227 = local read "T_PH_surf2"() -> (w358:dbl)
        n228 = local read "T_PH_surf3"() -> (w351:dbl)
        n229 = local read "G (kg/m²s)"() -> (w356:dbl)
        n230 = Build Array(w357, w358, w351, w352) -> (w359:dbl[])
        n231 = Greater Or Equal?(x="G minimum (kg/m²s)", y=w356) -> (x >= y?=w353:bool)
        "Mass alert" <- w353
        n232 = Array Max & Min(array=w359) -> (max value=w360:dbl)  [unwired: 3 out]
        "Temp max PH" <- w360
        n233 = Greater Or Equal?(x=w360, y="T limit PH (C)") -> (x >= y?=w355:bool)
        "Warning_TEMP" <- w355
        n234 = Or(x=w353, y=w355) -> (x .or. y?=w354:bool)
        n235 = case shown="True" w354 {
          tunnel: w364 -> [w376 w380]
          tunnel: w363 -> [w375 w379]
          tunnel: [w376 w378] -> w362
          tunnel: [w375 w377] -> w361
          frame False {
          }
          frame True {
            w382 = FALSE ("Power")
            w381 = 0.0 ("U Level")
            n236 = local write "Power PH"(w382) -> ()
            n237 = local write "U Level PH"(w381) -> ()
            n238 = call "Configure Output.vi"("error in (no error)"=w379, "Voltage Level (0.00 V)"=w381, "Enable Output (T: Enable)"=w382, "VISA resource name"=w380) -> ("error out"=w377:errorcluster, "VISA resource name out"=w378:refnum<visa-resource-name>)  [unwired: 5 in, 1 out]
          }
        }
        n239 = call "Read Output.vi"("error in (no error)"=w361, "VISA resource name"=w362) -> ("error out"=w371:errorcluster, "Actual Current Level (A)"=w367:dbl, "Actual Voltage Level (V)"=w368:dbl, "VISA resource name out"=w374:refnum<visa-resource-name>)  [unwired: 4 in, 2 out]
        "Actual Voltage Level (V) PH" <- w368
        "Actual Current Level (A) PH" <- w367
        n240 = Unbundle By Name(w371) -> ("status"=w370:bool)
        n241 = Multiply(x=w368, y=w367) -> (x*y=→"Power_PRE HEATER (W)":dbl)
        n242 = Not(x=w370) -> (.not. x?=→"Status DCS":bool)
      }
      frame "Stop" {
        w383 = FALSE ("Enable Output (T: Enable)")
        n243 = local write "Power PH"(w383) -> ()
        n244 = local write "Booléen"(w383) -> ()
        n245 = call "Configure Output.vi"("error in (no error)"=w387, "Voltage Level (0.00 V)"=0.0, "Enable Output (T: Enable)"=w383, "VISA resource name"=w388) -> ("error out"=w384:errorcluster, "VISA resource name out"=w385:refnum<visa-resource-name>)  [unwired: 5 in, 1 out]
        n246 = VISA Close(VISA resource name=w385, error in (no error)=w384) -> (error out=w389:errorcluster)
      }
      frame "Init" {
        w409 = u16 10 items=["1,0"=10, "1,5"=15, "2,0"=20] ("stop bits (10: 1 bit)")
        w408 = u16 0 items=["Aucun", "XON/XOFF", "RTS/CTS", "XON/XOFF & RTS/CTS", "DTR/DSR", "XON/XOFF & DTR/DSR"] ("flow control (0:none)")
        n247 = Concatenate Strings("*IDN?", "\r") -> (w407:string)
        n248 = call-poly "VISA Configure Serial Port"("VISA resource name"=w397, "timeout (10sec)"=u32 2000, "termination char\n(0xA = '\\n' = LF)"=u8 13 ("termination char\n(0xA = '\\n' = LF)"), "Enable Termination\nChar (T)"=TRUE ("Enable Termination\nChar (T)"), "baud rate (9600)"=u32 19200, "data bits (8)"=u16 8, "parity (0:none)"=enum16{"None", "Odd", "Even", "Mark", "Space"}."None", "error in (no error)"=w396, "stop bits (10: 1 bit)"=w409, "flow control (0:none)"=w408) -> ("VISA resource name out"=w401:refnum<visa-resource-name>, "error out"=w400:errorcluster)  [unwired: 4 in]
        n249 = VISA Write(VISA resource name=w401, write buffer=w407, error in (no error)=w400) -> (VISA resource name out=w405:refnum<visa-resource-name>, error out=w406:errorcluster)  [unwired: 1 out]
        n250 = VISA Read(VISA resource name=w405, byte count=u32 256 ("nombre d'octets"), error in (no error)=w406) -> (VISA resource name out=w399:refnum<visa-resource-name>, read buffer=→"Message":string, error out=w398:errorcluster)  [unwired: 1 out]
      }
      frame "WaitForEvent" {
        n251 = event shown="[1] Timeout" {
          selector: _ -> [_ _ _ _]
          dyn-events: _ -> [_ _ _ _]
          timeout: 50 -> [_ _ _ _]
          tunnel: [Commande."Power ON/OFF" Commande."Meas" Commande."Stop" Commande."Limit U&I"] -> w419
          event "Power PH", "U Level PH": Value Change {
            n252 = event-data() -> ()  [unwired: 1 in, 6 out]
          }
          event Timeout {
            n253 = event-data() -> ()  [unwired: 1 in, 3 out]
          }
          event "STOP PH": Value Change {
            n254 = event-data() -> ()  [unwired: 1 in, 6 out]
          }
          event "U limit PH", "I Limit PH": Value Change {
            n255 = event-data() -> ()  [unwired: 1 in, 6 out]
          }
        }
      }
      frame "Power ON/OFF" {
        n256 = call "Configure Output.vi"("error in (no error)"=w430, "Voltage Level (0.00 V)"="U Level PH", "Enable Output (T: Enable)"=w425, "VISA resource name"=w431) -> ("error out"=w428:errorcluster, "VISA resource name out"=w429:refnum<visa-resource-name>)  [unwired: 5 in, 1 out]
      }
    }
    "error out" <- w336
    "Booléen" <- "Power PH"
  }
  n257 = while {
    shift-right: [w438] -> _
    shift-left: w3 -> [w439]
    shift-right: [w437] -> _
    shift-left: refnum<visa-resource-name> "ASRL5::INSTR" ("VISA resource name") -> [w435]
    shift-right: [w436] -> _
    shift-left: errorcluster {"status"=FALSE, "code"=0, "source"=""} ("error out") -> [w434]
    tunnel: [w433] -> _
    stop <- w433 stop-if-true
    n258 = case shown="\"Meas\"" w439 {
      tunnel: [FALSE FALSE TRUE FALSE FALSE FALSE] -> w433
      tunnel: [Commande."WaitForEvent" Commande."WaitForEvent" Commande."Stop" Commande."Limit U&I" w526 Commande."WaitForEvent"] -> w438
      tunnel: [w442 w481 w492 w507 w523 w536] -> w437
      tunnel: [w441 w478 w496 w506 w524 w535] -> w436
      tunnel: w435 -> [w449 w471 w495 w505 w523 w538]
      tunnel: w434 -> [w448 w470 w494 w504 w524 w537]
      tunnel: "Power TS" -> [_ _ _ _ _ w532]
      frame "Limit U&I", Default {
        n259 = call "Configure Current Limit.vi"("error in (no error)"=w448, "Current Limit (0.00 A)"="I Limit TS", "VISA resource name"=w449) -> ("error out"=w443:errorcluster, "VISA resource name out"=w444:refnum<visa-resource-name>)  [unwired: 6 in, 1 out]
        n260 = call "Configure OVP.vi"("error in (no error)"=w443, "Overvoltage Protection Value (110.0 V)"="U limit TS", "VISA resource name"=w444) -> ("error out"=w441:errorcluster, "VISA resource name out"=w442:refnum<visa-resource-name>)  [unwired: 7 in]
      }
      frame "Meas" {
        # "Security system - 0 flow"
        # "Security system-Temperature"
        n261 = local read "TCHF_bot"() -> (w451:dbl)
        n262 = local read "TCHF_top"() -> (w450:dbl)
        n263 = local read "T1_mid"() -> (w465:dbl)
        n264 = local read "T1_bot"() -> (w464:dbl)
        n265 = local read "T2_mid"() -> (w456:dbl)
        n266 = local read "T1_top"() -> (w458:dbl)
        n267 = local read "T3_bot"() -> (w454:dbl)
        n268 = local read "G (kg/m²s)"() -> (w463:dbl)
        n269 = local read "T2_bot"() -> (w459:dbl)
        n270 = local read "T3_mid"() -> (w453:dbl)
        n271 = local read "T3_top"() -> (w452:dbl)
        n272 = local read "T2_top"() -> (w455:dbl)
        n273 = local read "G minimum (kg/m²s)"() -> (w457:dbl)
        n274 = Build Array(w464, w465, w458, w459, w456, w455, w454, w453, w452, w451, w450) -> (w466:dbl[])
        n275 = Greater Or Equal?(x=w457, y=w463) -> (x >= y?=w460:bool)
        n276 = Array Max & Min(array=w466) -> (max value=w467:dbl)  [unwired: 3 out]
        "Temp max TS" <- w467
        n277 = Greater Or Equal?(x=w467, y="T limit_TS (C)") -> (x >= y?=w462:bool)
        "Warning_Temp_TS" <- w462
        n278 = Or(x=w460, y=w462) -> (x .or. y?=w461:bool)
        n279 = case shown="True" w461 {
          tunnel: w471 -> [w483 w487]
          tunnel: w470 -> [w482 w486]
          tunnel: [w483 w485] -> w469
          tunnel: [w482 w484] -> w468
          frame False {
          }
          frame True {
            w489 = FALSE ("Power")
            w488 = 0.0 ("U Level")
            n280 = local write "Power TS"(w489) -> ()
            n281 = local write "U Level TS"(w488) -> ()
            n282 = call "Configure Output.vi"("error in (no error)"=w486, "Voltage Level (0.00 V)"=w488, "Enable Output (T: Enable)"=w489, "VISA resource name"=w487) -> ("error out"=w484:errorcluster, "VISA resource name out"=w485:refnum<visa-resource-name>)  [unwired: 5 in, 1 out]
          }
        }
        n283 = call "Read Output.vi"("error in (no error)"=w468, "VISA resource name"=w469) -> ("error out"=w478:errorcluster, "Actual Current Level (A)"=w474:dbl, "Actual Voltage Level (V)"=w475:dbl, "VISA resource name out"=w481:refnum<visa-resource-name>)  [unwired: 4 in, 2 out]
        "Actual Voltage Level (V) TS" <- w475
        "Actual Current Level (A) TS" <- w474
        n284 = Unbundle By Name(w478) -> ("status"=w477:bool)
        n285 = Multiply(x=w475, y=w474) -> (x*y=→"Power_Test section (W)":dbl)
        n286 = Not(x=w477) -> (.not. x?=→"status SGA":bool)
      }
      frame "Stop" {
        w490 = FALSE ("Enable Output (T: Enable)")
        n287 = local write "Power TS"(w490) -> ()
        n288 = local write "Booléen 2"(w490) -> ()
        n289 = call "Configure Output.vi"("error in (no error)"=w494, "Voltage Level (0.00 V)"=0.0, "Enable Output (T: Enable)"=w490, "VISA resource name"=w495) -> ("error out"=w491:errorcluster, "VISA resource name out"=w492:refnum<visa-resource-name>)  [unwired: 5 in, 1 out]
        n290 = VISA Close(VISA resource name=w492, error in (no error)=w491) -> (error out=w496:errorcluster)
      }
      frame "Init" {
        w517 = u16 10 items=["1,0"=10, "1,5"=15, "2,0"=20] ("stop bits (10: 1 bit)")
        w516 = u16 0 items=["Aucun", "XON/XOFF", "RTS/CTS", "XON/XOFF & RTS/CTS", "DTR/DSR", "XON/XOFF & DTR/DSR"] ("flow control (0:none)")
        n291 = Concatenate Strings("*IDN?", "\r") -> (w515:string)
        n292 = call-poly "VISA Configure Serial Port"("VISA resource name"=w505, "timeout (10sec)"=u32 2000, "termination char\n(0xA = '\\n' = LF)"=u8 10 ("termination char\n(0xA = '\\n' = LF)"), "Enable Termination\nChar (T)"=TRUE ("Enable Termination\nChar (T)"), "baud rate (9600)"=u32 19200, "data bits (8)"=u16 8, "parity (0:none)"=enum16{"None", "Odd", "Even", "Mark", "Space"}."None", "error in (no error)"=w504, "stop bits (10: 1 bit)"=w517, "flow control (0:none)"=w516) -> ("VISA resource name out"=w509:refnum<visa-resource-name>, "error out"=w508:errorcluster)  [unwired: 4 in]
        n293 = VISA Write(VISA resource name=w509, write buffer=w515, error in (no error)=w508) -> (VISA resource name out=w513:refnum<visa-resource-name>, error out=w514:errorcluster)  [unwired: 1 out]
        n294 = VISA Read(VISA resource name=w513, byte count=u32 256 ("nombre d'octets"), error in (no error)=w514) -> (VISA resource name out=w507:refnum<visa-resource-name>, read buffer=→"Message 2":string, error out=w506:errorcluster)  [unwired: 1 out]
      }
      frame "WaitForEvent" {
        n295 = event shown="[3] \"U limit TS\", \"I Limit TS\": Value Change" {
          selector: _ -> [_ _ _ _]
          dyn-events: _ -> [_ _ _ _]
          timeout: 50 -> [_ _ _ _]
          tunnel: [Commande."Power ON/OFF" Commande."Meas" Commande."Stop" Commande."Limit U&I"] -> w526
          event "Power TS", "U Level TS": Value Change {
            n296 = event-data() -> ()  [unwired: 1 in, 6 out]
          }
          event Timeout {
            n297 = event-data() -> ()  [unwired: 1 in, 3 out]
          }
          event "STOP TS": Value Change {
            n298 = event-data() -> ()  [unwired: 1 in, 6 out]
          }
          event "U limit TS", "I Limit TS": Value Change {
            n299 = event-data() -> ()  [unwired: 1 in, 6 out]
          }
        }
      }
      frame "Power ON/OFF" {
        n300 = call "Configure Output.vi"("error in (no error)"=w537, "Voltage Level (0.00 V)"="U Level TS", "Enable Output (T: Enable)"=w532, "VISA resource name"=w538) -> ("error out"=w535:errorcluster, "VISA resource name out"=w536:refnum<visa-resource-name>)  [unwired: 5 in, 1 out]
      }
    }
    "error out 2" <- w436
    "Booléen 2" <- "Power TS"
  }
  n301 = call <instrlib>:"Close.vi"("VISA resource name"=w11, "error in (no error)"=w10) -> ()  [unwired: 13 in, 1 out]
  n302 = Compound Arithmetic op=AND(w7, w6) -> (w5:bool)
  n303 = Not(x=w5) -> (.not. x?=w53:bool)
  n304 = local write "stop"(w53) -> ()
  n305 = local write "stop flag"(w53) -> ()
